vi "运行批处理.vi"   [LabVIEW 2011]
types:
  T1 = enum16{"open", "replace", "create", "open or create", "replace or create", "replace or create with confirmation"}
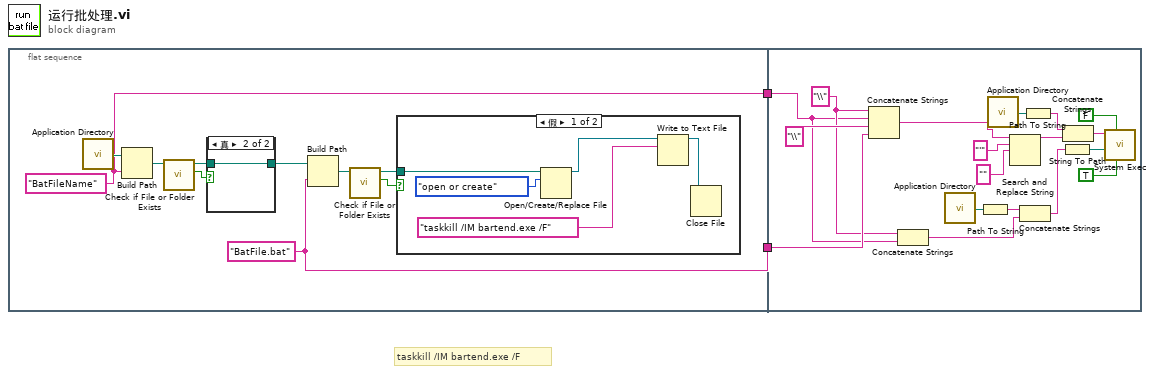
[diagram p0: block diagram]
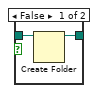
[diagram p3: hidden frame]
diagram:
  # "taskkill /IM bartend.exe /F"
  n1 = flat-sequence {
    tunnel: [w4] -> w2
    tunnel: [w3] -> w1
    tunnel: w2 -> [w22]
    tunnel: w1 -> [w25]
    frame #0 {
      w3 = "BatFile.bat" ("名称或相对路径")
      w4 = "BatFileName" ("名称或相对路径")
      n2 = call <vilib>:"Application Directory.vi"() -> ("Application Directory"=w5:path)
      n3 = Build Path(base path=w5, name or relative path=w4) -> (appended path=w6:path)
      n4 = call <vilib>:"Check if File or Folder Exists.vi"("path"=w6) -> ("file or folder exists?"=w7:bool, "dup path"=w8:path)  [unwired: 8 in, 1 out]
      n5 = case shown="真" w7 {
        tunnel: w8 -> [w19 w20]
        tunnel: [w18 w20] -> w9
        frame False {
          n6 = Create Folder(path (use dialog)=w19) -> (created path=w18:path)  [unwired: 2 in, 2 out]
        }
        frame True {
        }
      }
      n7 = Build Path(base path=w9, name or relative path=w3) -> (appended path=w10:path)
      n8 = call <vilib>:"Check if File or Folder Exists.vi"("path"=w10) -> ("file or folder exists?"=w11:bool, "dup path"=w12:path)  [unwired: 8 in, 1 out]
      n9 = case shown="假" w11 {
        tunnel: w12 -> [w17 _]
        frame False {
          n10 = Open/Create/Replace File(file path (use dialog)=w17, operation (0:open)=T1."open or create" ("操作(0:open)")) -> (refnum out=w15:refnum<file>)  [unwired: 4 in, 2 out]
          n11 = Write to Text File(file (use dialog)=w15, text="taskkill /IM bartend.exe /F" ("文本")) -> (refnum out=w13:refnum<file>)  [unwired: 2 in, 2 out]
          n12 = Close File(refnum=w13) -> ()  [unwired: 1 in, 2 out]
        }
        frame True {
        }
      }
    }
    frame #1 {
      w23 = "\\" ("字符串")
      n13 = Concatenate Strings(w23, w22, "\\" ("字符串"), w25) -> (w24:string)
      n14 = Concatenate Strings(w23, w22) -> (w21:string)
      n15 = call <vilib>:"Application Directory.vi"() -> ("Application Directory"=w30:path)
      n16 = Path To String(path=w30) -> (string=w31:string)
      n17 = call <vilib>:"Application Directory.vi"() -> ("Application Directory"=w27:path)
      n18 = Search and Replace String(input string=w24, search string="'" ("搜索字符串"), replace string="" ("替换字符串(\"\")")) -> (result string=w36:string)  [unwired: 5 in, 3 out]
      n19 = Concatenate Strings(w31, w21) -> (w37:string)
      n20 = Path To String(path=w27) -> (string=w28:string)
      n21 = String To Path(string=w37) -> (path=w38:path)
      n22 = Concatenate Strings(w28, w36) -> (w29:string)
      n23 = call <vilib>:"System Exec.vi"("run minimized? (F)"=TRUE, "wait until completion? (T)"=FALSE, "working directory"=w38, "command line"=w29) -> ()  [unwired: 4 in, 4 out]
    }
  }
